vi "ListenForSubscriber.vi"(2 "LogPath in":path, 3 "ROS":T1) -> (0 "heard?":errorcluster, 1 "server":refnum<k5>)   [LabVIEW 2012]
doc: "Listens on the TCP network for a subscriber"
uses:
  <userlib>/ROS for LabVIEW Software/ROS/Code/SubVIs/_ROSControl.ctl
  <userlib>/ROS for LabVIEW Software/ROS/Code/SubVIs/_ROSDirection.ctl
  <userlib>/ROS for LabVIEW Software/ROS/Code/Console/Servers/ServerSubs/MyState.ctl
  <userlib>/ROS for LabVIEW Software/ROS/Code/_ROSDefinition.vi
panel:
  out "LogPath out":path
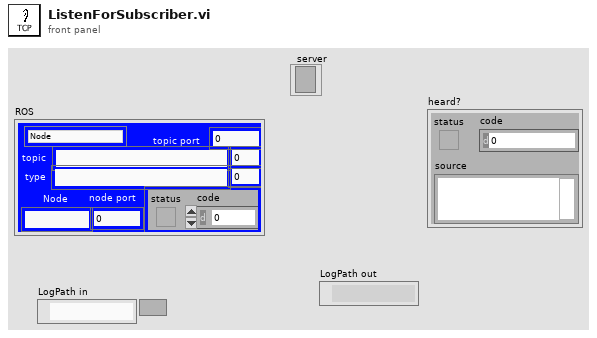
[diagram p1: front panel]
types:
  T1 = typedef "_ROSControl.ctl" = cluster{"topic port":u16, "Node":string, "topic":string, "type":string, "node port":u16, "error ":errorcluster, "Direction":T2, "Update (ms)":u16, "FIFO size":u16}
  T2 = typedef "_ROSDirection.ctl" = enum16{"Node", "Publisher", "Subscriber", "ServiceClient", "ServiceProvider"}
  T3 = typedef "MyState.ctl" = enum16{"No Connection", "Registered", "Connected", "Close"}
  T4 = typedef "ROSLog.ctl" = cluster{"Sent":string, "Reply":string, "MethodName":string, "success":bool, "Dir1":string, "Dir2":string, "Time Stamp":string, "error":errorcluster, "Preamble":string, "Midamble":string, "Postamble":string}
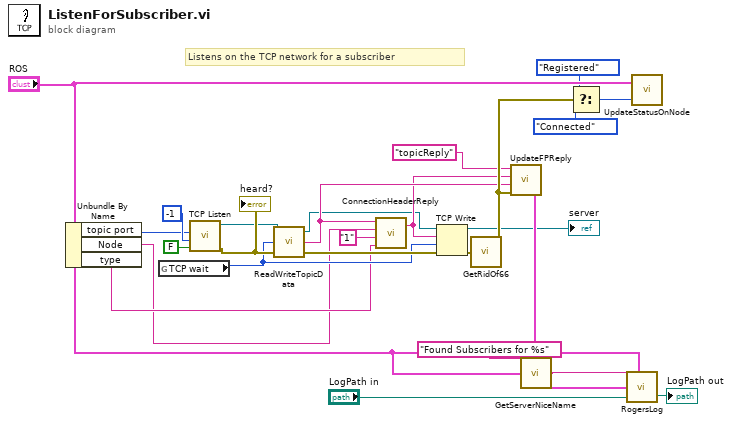
[diagram p0: block diagram]
diagram:
  # "Listens on the TCP network for a subscriber"
  n1 = Unbundle By Name("ROS") -> ("topic port"=w3:u16, "Node"=w4:string, "type"=w5:string)
  n2 = global read "_ROSDefinition.vi" "TCP wait"() -> (w6:i32)
  n3 = call <vilib>:"TCP Listen.vi"("resolve remote address (T)"=FALSE, "timeout ms (wait forever: -1)"=-1, "port"=w3) -> ("error out"=w7:errorcluster, "connection ID"=w1:refnum<k5>)  [unwired: 4 in, 3 out]
  "heard?" <- w7
  n4 = call <userlib>:"ReadWriteTopicData.vi"("error in (no error)"=w7, "timeout ms (1000)"=w6, "connection ID in"=w1) -> ("error out"=w11:errorcluster, "data out"=w13:string, "connection ID out"=w10:refnum<k5>)
  n5 = call <userlib>:"ConnectionHeaderReply.vi"("type"=w5, "Latching"="1", "Caller ID"=w4, "TCPROS Connection Header"=w13) -> ("Connection Response"=w12:string)  [unwired: 1 in]
  n6 = TCP Write(connection ID=w10, data in=w12, error in (no error)=w11, 9:w6) -> (connection ID out=→"server":refnum<k5>, error out=w16:errorcluster)  [unwired: 1 out]
  n7 = call <userlib>:"GetRidOf66.vi"("error in (no error)"=w16) -> ("error out"=w18:errorcluster)
  n8 = call <userlib>:"UpdateFPReply.vi"("error in (no error)"=w18, "Reply"=w13, "Sent"=w12, "method"="topicReply") -> ("Log"=w20:T4)
  n9 = call <userlib>:"GetServerNiceName.vi"("ROS"="ROS", "Text to add"="Found Subscribers for %s") -> ("String"=w23:string)
  n10 = Select(t=MyState."Registered" ("MyState"), s=w18, f=MyState."Connected" ("MyState")) -> (s? t:f=w25:T3)
  n11 = call <userlib>:"RogersLog.vi"("Text to add"=w23, "ROS"="ROS", "Log"=w20, "LogPath in"="LogPath in") -> ("LogPath out"=→"LogPath out":path)  [unwired: 1 in, 1 out]
  n12 = call <userlib>:"UpdateStatusOnNode.vi"("MyState"=w25, "ROS"="ROS") -> ()  [unwired: 1 in, 1 out]
